vi "send frame rate.vi"(8 "error in (no error)":errorcluster, 11 "Waveform in":refnum<class "Waveform.lvclass">) -> (0 "error out":errorcluster, 3 "Waveform out":refnum<class "Waveform.lvclass">)   [LabVIEW 2012, in "Waveform.lvclass"]
uses:
  Waveform.lvclass
  Waveform.lvclass/Waveform.ctl
  <vilib>/Distrio/Murmex/Murmex/update_cluster.ctl
  <vilib>/Distrio/Murmex/Murmex/Murmex.lvclass
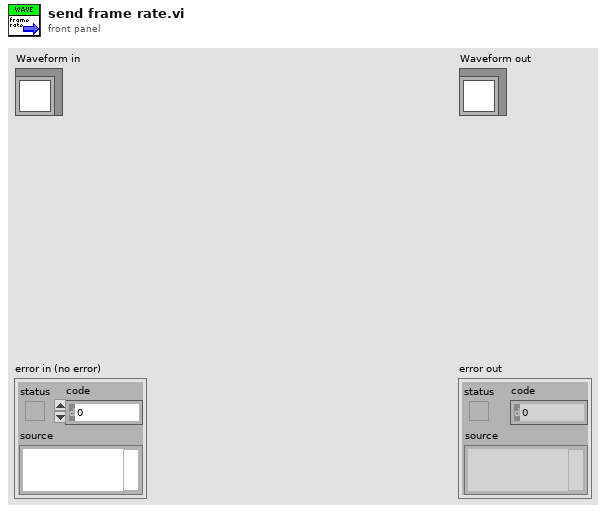
[diagram p1: front panel]
types:
  T1 = typedef "Murmex.lvlib/Murmex.lvclass/update_cluster.ctl" = cluster{"target ID":string, "key chains":string[], "values":variant[]}
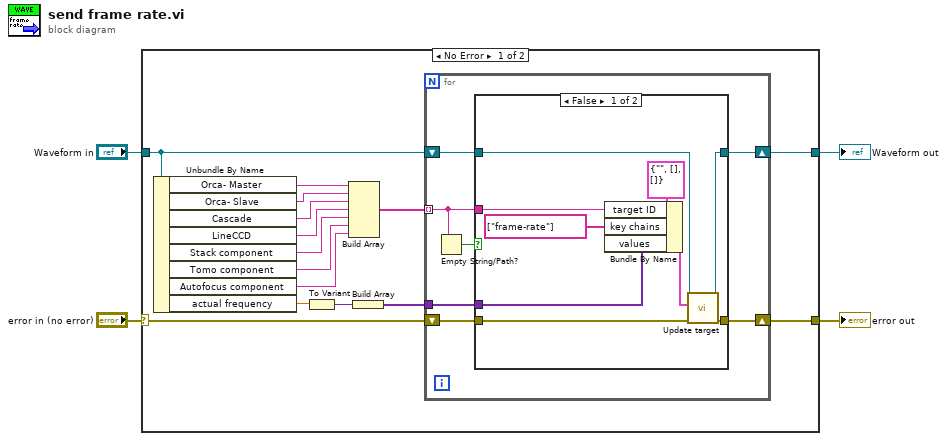
[diagram p0: block diagram]
diagram:
  n1 = case shown="No Error" "error in (no error)" {
    selector: "error in (no error)" -> [w8 w39]
    tunnel: [w7 w39] -> w3
    tunnel: [w9 w38] -> w1
    tunnel: "Waveform in" -> [w10 w38]
    frame No Error {
      n2 = Unbundle By Name(w10) -> ("Orca- Master"=w19:string, "Orca- Slave"=w18:string, "Cascade"=w17:string, "LineCCD"=w16:string, "Stack component"=w15:string, "Tomo component"=w14:string, "Autofocus component"=w13:string, "actual frequency"=w12:dbl[unit])
      n3 = To Variant(anything=w12) -> (Variant=w11:variant)
      n4 = Build Array(w19, w18, w17, w16, w15, w14, w13) -> (w6:string[])
      n5 = Build Array(w11) -> (w5:variant[])
      n6 = for {
        shift-right: [w23] -> w9
        shift-left: w10 -> [w24]
        shift-right: [w25] -> w7
        shift-left: w8 -> [w26]
        tunnel: w6 -> [w21] mode=indexing
        tunnel: w5 -> [w20]
        n7 = Empty String/Path?(string/path=w21) -> (empty?=w22:bool)
        n8 = case shown="False" w22 {
          tunnel: [w34 w36] -> w25
          tunnel: w26 -> [w35 w36]
          tunnel: w24 -> [w32 w37]
          tunnel: [w31 w37] -> w23
          tunnel: w21 -> [w30 _]
          tunnel: w20 -> [w28 _]
          frame False {
            n9 = Bundle By Name(cluster=T1 {"target ID"="", "key chains"=[], "values"=[]} ("update cluster"), "target ID"=w30, "key chains"=string[] ["frame-rate"], "values"=w28) -> (w29:T1)
            n10 = call <vilib>:"Update target.vi"("error in (no error)"=w35, "update cluster"=w29, "MurmexBase in"=w32) -> ("error out"=w34:errorcluster, "MurmexBase out"=w31:refnum<class "Waveform.lvclass">)  [unwired: 7 in]
          }
          frame True {
          }
        }
      }
    }
    frame Error {
    }
  }
  "error out" <- w3
  "Waveform out" <- w1
